vi "ENA_SettingMeas_Markers.vi"(4 "Mark_Freq(GHz)":dbl=39.0, 5 "Stop_Freq(GHz)":dbl=31.5, 7 "Start_Freq(GHz)":dbl=26.5, 8 "error in":errorcluster, 9 "sParameter":i32=21, 10 "Step_Freq(GHz)":dbl=0.5 format="%#_13g", 11 "VISA IN":refnum<visa-resource-name>="TCPIP0::192.168.100.12::inst0::INSTR") -> (0 "error out":errorcluster, 3 "Marker_array":dbl[](array[numeric]))   [LabVIEW 2023, in "Keysight.lvlib"]
uses:
  Keysight.lvlib
  CTL/Keysight_VNA.ctl
panel:
  out "output cluster":T1
  in  "Mark":i32=1
  in  "Meas":i32=1
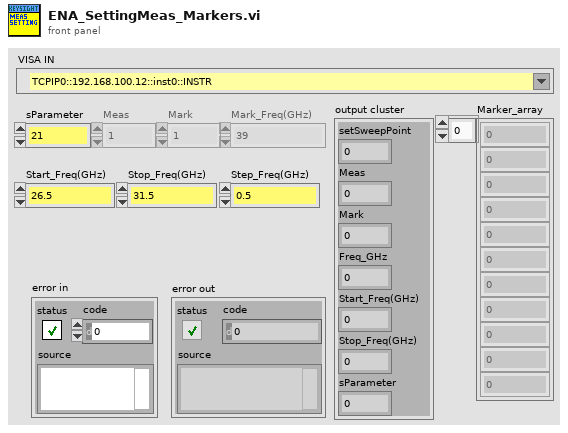
[diagram p1: front panel]
types:
  T1 = cluster{"setSweepPoint":i32, "Meas":i32, "Mark":i32, "Freq_GHz":dbl, "Start_Freq(GHz)":dbl, "Stop_Freq(GHz)":dbl, "sParameter":i32}
  T2 = typedef "Keysight_VNA.ctl" = enum16{"Init", "queryMarker", "setSweepPoint", "setMarkerFreq", "setMeasureFormat", "setFreqStartStop", "setMarkerOnOFF", "setMarkerFormat_LOGP", "setMeasPAR_S", "setTriggerSingle", "Trigger_Save_SnP", "Trigger_Single", "Close"}
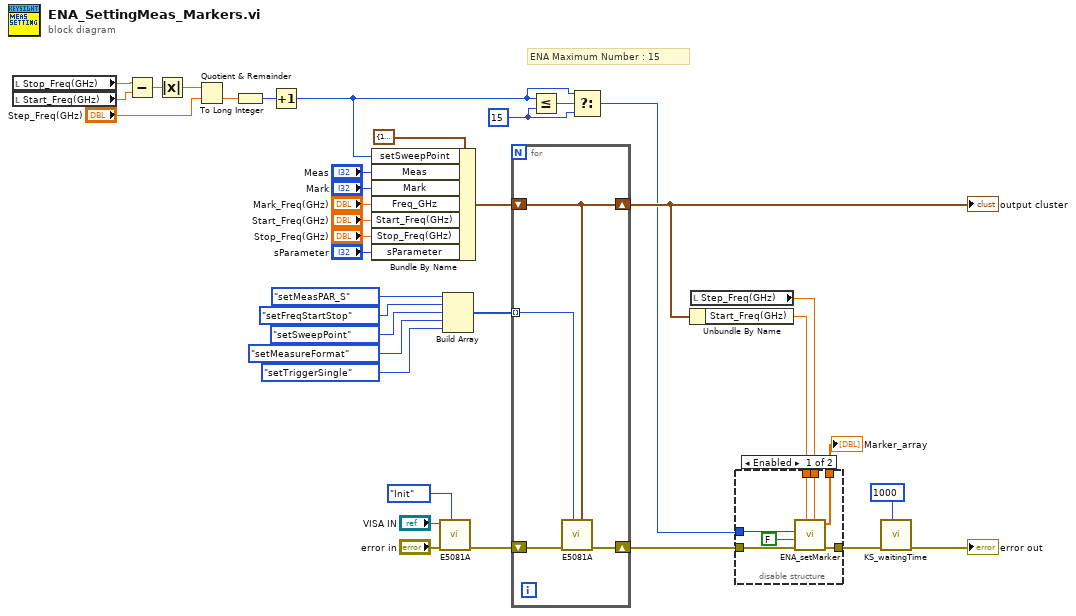
[diagram p0: block diagram]
diagram:
  w4 = 15 ("y")
  # "ENA Maximum Number : 15"
  n1 = local read "Stop_Freq(GHz)"() -> (w27:dbl)
  n2 = local read "Start_Freq(GHz)"() -> (w26:dbl)
  n3 = Subtract(x=w27, y=w26) -> (x-y=w25:dbl)
  n4 = Absolute Value(x=w25) -> (abs(x)=w23:dbl)
  n5 = Quotient & Remainder(x=w23, y="Step_Freq(GHz)") -> (floor(x/y)=w22:dbl)  [unwired: 1 out]
  n6 = To Long Integer(number=w22) -> (32bit integer=w21:i32)
  n7 = Increment(x=w21) -> (x+1=w1:i32)
  n8 = Bundle By Name(cluster=T1 {"setSweepPoint"=11, "Meas"=1, "Mark"=0, "Freq_GHz"=0.0, "Start_Freq(GHz)"=0.0, "Stop_Freq(GHz)"=0.0, "sParameter"=1} ("Input"), "setSweepPoint"=w1, "Meas"="Meas", "Mark"="Mark", "Freq_GHz"="Mark_Freq(GHz)", "Start_Freq(GHz)"="Start_Freq(GHz)", "Stop_Freq(GHz)"="Stop_Freq(GHz)", "sParameter"="sParameter") -> (w20:T1)
  n9 = call "E5081A.vi"("Function_VNA"=Keysight_VNA."Init", "error in"="error in", "VISA IN"="VISA IN") -> ("error out"=w35:errorcluster)  [unwired: 7 in, 1 out]
  n10 = Build Array(Keysight_VNA."setMeasPAR_S" ("Function_VNA"), Keysight_VNA."setFreqStartStop" ("Function_VNA"), Keysight_VNA."setSweepPoint" ("Function_VNA"), Keysight_VNA."setMeasureFormat" ("Function_VNA"), Keysight_VNA."setTriggerSingle" ("Function_VNA")) -> (w14:T2[])
  n11 = for {
    shift-right: [w40] -> w10
    shift-left: w20 -> [w40]
    tunnel: w14 -> [w39] mode=indexing
    shift-right: [w38] -> w13
    shift-left: w35 -> [w41]
    n12 = call "E5081A.vi"("Input"=w40, "Function_VNA"=w39, "error in"=w41) -> ("error out"=w38:errorcluster)  [unwired: 7 in, 1 out]
  }
  "output cluster" <- w10
  n13 = Less Or Equal?(x=w1, y=w4) -> (x <= y?=w5:bool)
  n14 = Select(t=w1, s=w5, f=w4) -> (s? t:f=w3:i32)
  n15 = Unbundle By Name(w10) -> ("Start_Freq(GHz)"=w12:dbl)
  n16 = local read "Step_Freq(GHz)"() -> (w11:dbl)
  n17 = disable-structure shown="Enabled" {
    disable-tunnel: w13 -> [w48 w49]
    disable-tunnel: w12 -> [w46 _]
    disable-tunnel: w11 -> [w45 _]
    disable-tunnel: [w44 w49] -> w9
    disable-tunnel: w3 -> [w43 _]
    disable-tunnel: [w42 _] -> w2
    frame Enabled {
      n18 = call "ENA_setMarker.vi"("Step_Freq(GHz)"=w45, "Start_Freq(GHz)"=w46, "error in"=w48, "Simulation"=FALSE, "Markers_num"=w43) -> ("error out"=w44:errorcluster, "Marker_array"=w42:dbl[])  [unwired: 5 in]
    }
    frame Disabled {
    }
  }
  "Marker_array" <- w2
  n19 = call "KS_waitingTime.vi"("Waiting Time(ms)"=u32 1000, "error in"=w9) -> ("error out"=→"error out":errorcluster)  [unwired: 9 in]
